vi "SanboxVAlveModbus.vi"() -> ()   [LabVIEW 2019]
uses:
  MB_ENGINE_class/Settings.ctl
  MB_ENGINE_class/Engine State.ctl
  MB_ENGINE_class/Engine Alarms.ctl
  TypeDef/StateValveModbus.ctl
  MB_ENGINE_class/cmd enum.ctl
  ValveModbus_class/ValveModbus.lvclass
  MB_ENGINE_class/MB_ENGINE.lvclass
  D:/H4000/src/modbus engine custom/MB_MODULE_class/MB_MODULE.lvclass
  ValveModbus_class/ValveModbus.lvclass/ValveModbus.ctl
  <vilib>/NI/Modbus Library/API/Wrapper/Create TCP Master.vi
  <vilib>/NI/Modbus Library/API/Wrapper/API Main.lvlib
  MB_MODULE_class/MB_MODULE.lvclass
panel:
  out "StateValveModbus 2":T1
  in  "delta pres":dbl=1.0
  in  "average":i32=10
  in  "ValveModbus":refnum<class "ValveModbus.lvclass">
  in  "milliseconds to wait":u32=300
  out "angle":dbl(graph)=3.4981473129739618
  out "encoder":i32(graph)=72974
  out "step":i32(graph)=124110
  in  "SET":bool
  in  "cmd to write":T2=20 items=["0 Idle"=0, "1 GoTo Absolute Position"=1, "2 GoTo Relative"=2, "10 GoTo Home Position"=10, "11 Set Home Position"=11, "12 Set FindHome Mode"=12, "13 Reset FindHome Mode"=13, "14 Get FindHome State"=14, "20 Hard Stop"=20, "21 HiZ Stop"=21, "22 Soft Stop"=22, "30 Clear Fault"=30, "40 Encoder Set Home"=40, "70 Driver Init"=70]
  out "StateValveModbus":T1
  in  "PRESSURE":dbl(slide)=4.7148288973384025 scale=0.0..10.0
  in  "stop_":bool
  in  "close":bool
  in  "open":bool
  out "dt":u32=10
  in  "cluster 2":T3={"ACC Steps Per Sec^2"=50, "DEC Steps Per Sec^2"=50, "Min Velosity Step Per Sec"=100, "Max Velosity Step Per Sec"=200, "MicroStep"=16}
  out "Numeric":i32=3223
  in  "stop":bool
  out "type":u16=1
  out "Alarms":T4={"OL"=FALSE, "TF"=FALSE, "STL"=FALSE, "OCP"=FALSE, "CPUV"=FALSE, "UVLO"=FALSE, "SPI_ERROR"=FALSE, "Fault"=FALSE, "OL 2"=FALSE, "TF 2"=FALSE, "STL 2"=FALSE, "OCP 2"=FALSE, "CPUV 2"=FALSE, "UVLO 2"=FALSE, "reserved"=TRUE, "InitDone"=TRUE}
  out "Engine State":T5=8 items=["ACCELERATING", "DECELERATINGTOSTOP", "DECELERATING", "STEADY", "INDEX_ACCEL", "NDEX_RUN", "INDEX_DECEL", "INDEX_DWELL", "INACTIVE", "STANDBY", "STANDBYTOINACTIVE"]
  out "RAW Possition":i32=124110
  out "cluster":T3={"ACC Steps Per Sec^2"=100, "DEC Steps Per Sec^2"=100, "Min Velosity Step Per Sec"=100, "Max Velosity Step Per Sec"=200, "MicroStep"=16}
  out "error out":errorcluster
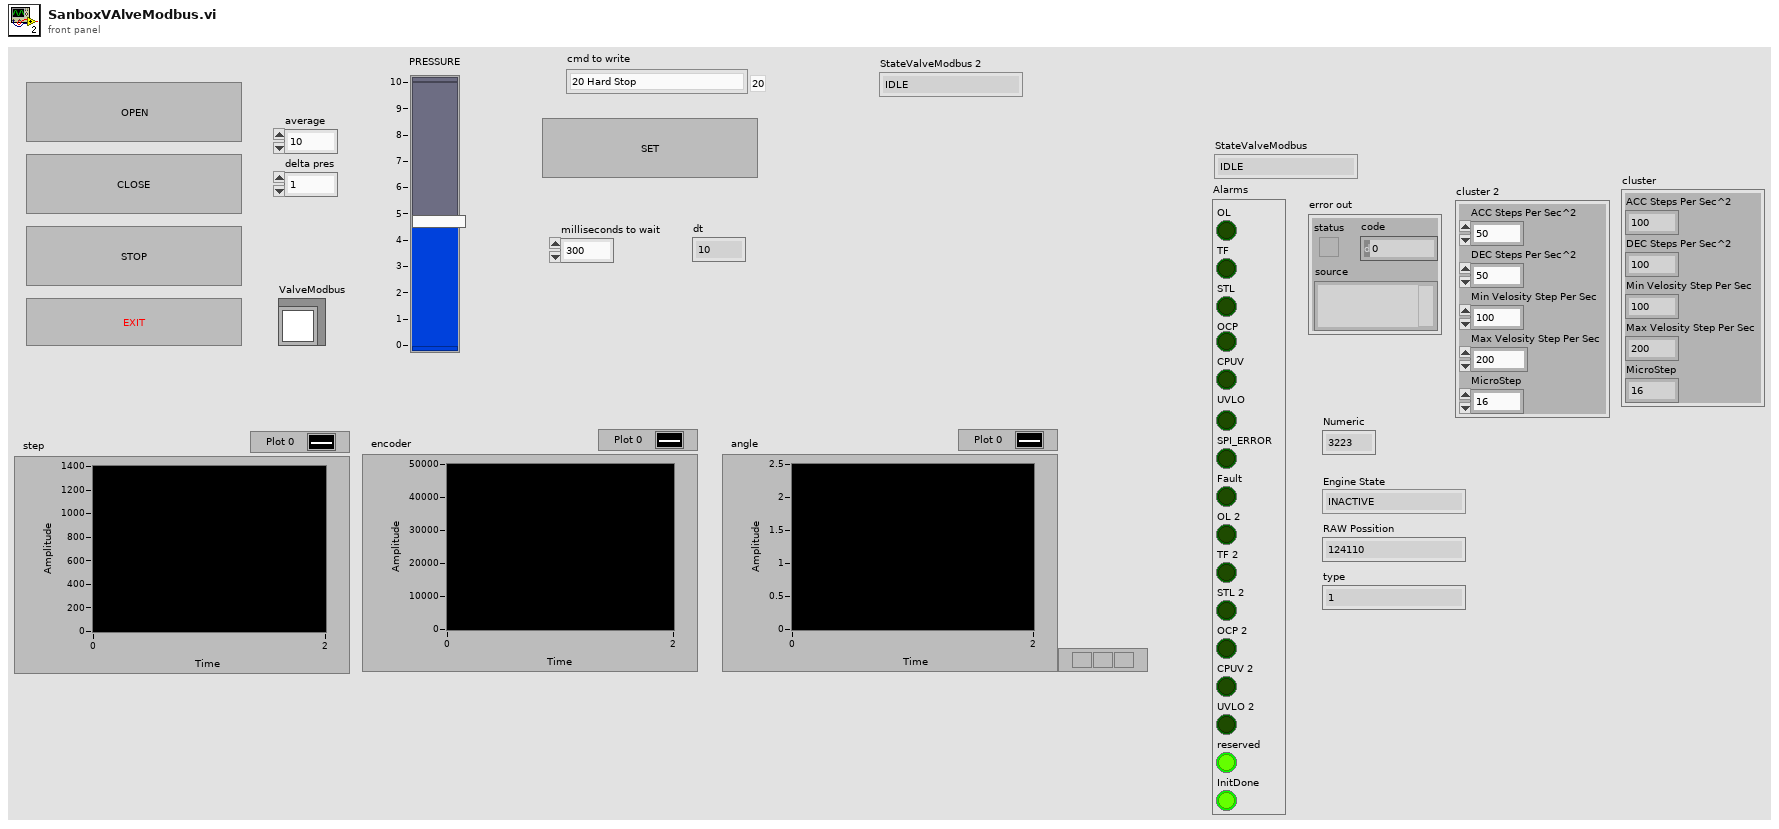
[diagram p1: front panel]
types:
  T1 = typedef "StateValveModbus.ctl" = enum16{"IDLE", "OPEN", "CLOSE", "OPENING", "CLOSING", "STOP"}
  T2 = typedef "MB_ENGINE.lvclass/cmd enum.ctl" = u16
  T3 = typedef "MB_ENGINE.lvclass/Settings.ctl" = cluster{"ACC Steps Per Sec^2":u16, "DEC Steps Per Sec^2":u16, "Min Velosity Step Per Sec":u16, "Max Velosity Step Per Sec":u16, "MicroStep":u16}
  T4 = typedef "MB_ENGINE.lvclass/Engine Alarms.ctl" = cluster{"OL":bool, "TF":bool, "STL":bool, "OCP":bool, "CPUV":bool, "UVLO":bool, "SPI_ERROR":bool, "Fault":bool, "OL 2":bool, "TF 2":bool, "STL 2":bool, "OCP 2":bool, "CPUV 2":bool, "UVLO 2":bool, "reserved":bool, "InitDone":bool}
  T5 = typedef "MB_ENGINE.lvclass/Engine State.ctl" = u16
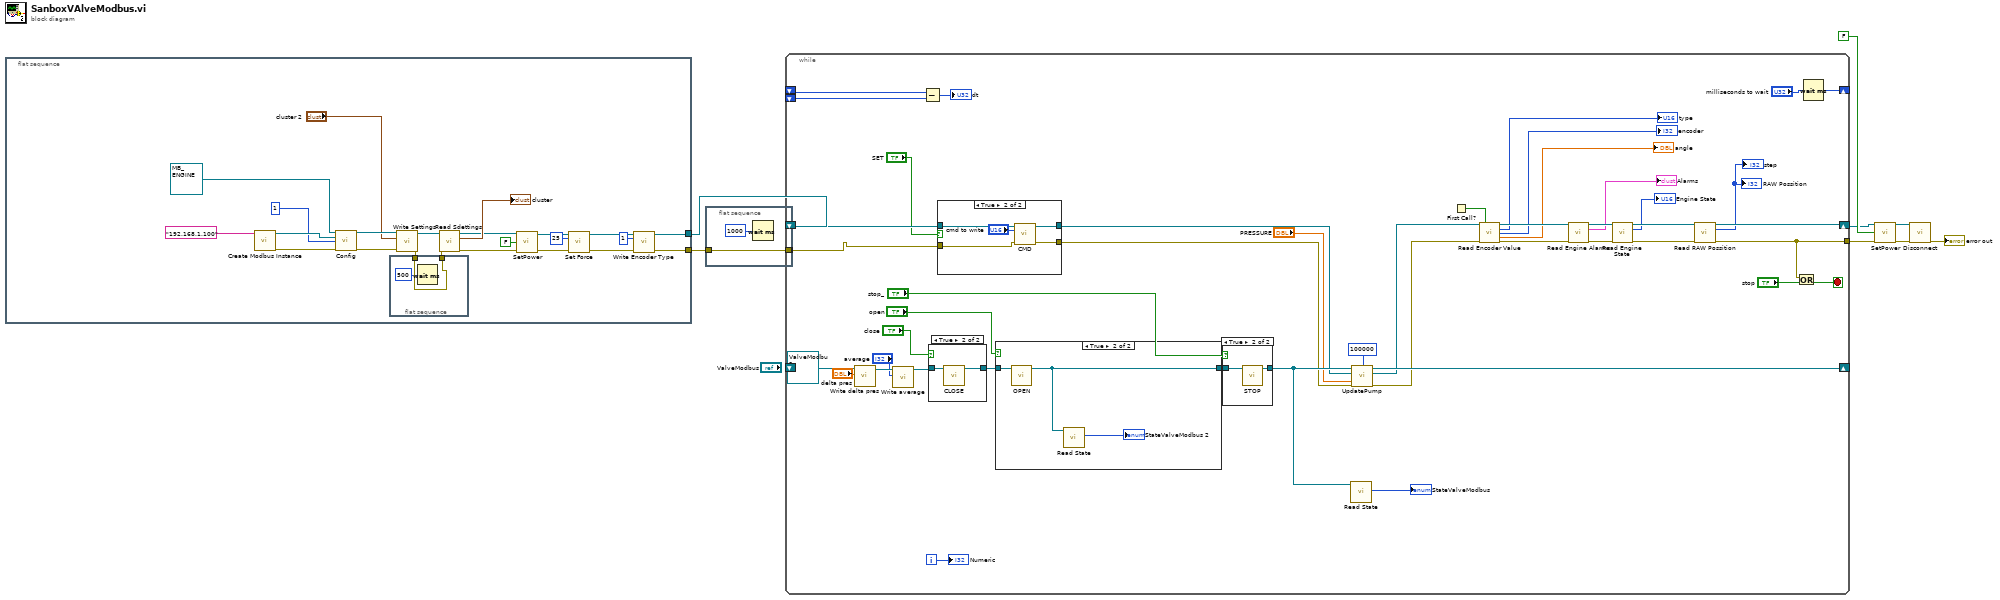
[diagram p0: block diagram]
diagram:
  n1 = flat-sequence {
    tunnel: [w14] -> w9
    tunnel: [w13] -> w2
    frame #0 {
      n2 = call-poly <vilib>:"Create Modbus Instance.vi"("address"="192.168.1.100") -> ("error out"=w30:errorcluster, "TCP master instance"=w32:refnum<class "Modbus Master.lvclass">)  [unwired: 9 in]
      n3 = call-dynamic "Config.vi"("class data in"=refnum<class "MB_ENGINE.lvclass"> refnum ("MB_ENGINE"), "modbus"=w32, "addres"=u16 1, "error in (no error)"=w30) -> ("class data out"=w27:refnum<class "MB_ENGINE.lvclass">, "error out"=w26:errorcluster)  [unwired: 10 in]
      n4 = flat-sequence {
        tunnel: [w35] -> w12
        tunnel: w11 -> [w35]
        frame #0 {
          n5 = Wait (ms)(milliseconds to wait=u32 500) -> ()  [unwired: 1 out]
        }
      }
      n6 = call-dynamic "Write Settings.vi"("class data in"=w27, "cluster"="cluster 2", "error in (no error)"=w26) -> ("class data out"=w24:refnum<class "MB_ENGINE.lvclass">, "error out"=w11:errorcluster)  [unwired: 11 in]
      n7 = call-dynamic "Read Sdettings.vi"("class data in"=w24, "error in (no error)"=w12) -> ("class data out"=w23:refnum<class "MB_ENGINE.lvclass">, "cluster"=→"cluster":T3, "error out"=w22:errorcluster)  [unwired: 11 in]
      n8 = call-dynamic "SetPower.vi"("class data in"=w23, "On"=FALSE, "error in (no error)"=w22) -> ("class data out"=w20:refnum<class "MB_ENGINE.lvclass">, "error out"=w19:errorcluster)  [unwired: 11 in]
      n9 = call-dynamic "Set Force.vi"("class data in"=w20, "percent"=u16 25, "error in (no error)"=w19) -> ("class data out"=w17:refnum<class "MB_ENGINE.lvclass">, "error out"=w16:errorcluster)  [unwired: 11 in]
      n10 = call-dynamic "Write Encoder Type.vi"("class data in"=w17, "U16"=u16 1, "error in (no error)"=w16) -> ("class data out"=w14:refnum<class "MB_ENGINE.lvclass">, "error out"=w13:errorcluster)  [unwired: 11 in]
    }
  }
  n11 = flat-sequence {
    tunnel: [w37] -> w1
    tunnel: w2 -> [w37]
    frame #0 {
      n12 = Wait (ms)(milliseconds to wait=u32 1000) -> ()  [unwired: 1 out]
    }
  }
  n13 = while {
    tunnel: [w76] -> w6
    shift-right: [w73] -> _
    shift-left: _ -> [w72]
    shift-left: _ -> [w71]
    shift-right: [w77] -> w7
    shift-left: w9 -> [w54]
    shift-right: [w60] -> _
    shift-left: refnum<class "ValveModbus.lvclass"> refnum ("ValveModbus") -> [w42]
    tunnel: w1 -> [w43]
    i -> [w75]
    stop <- w78 stop-if-true
    n14 = call "Write delta pres.vi"("delta pres"="delta pres", "ValveModbus in"=w42) -> ("ValveModbus out"=w41:refnum<class "ValveModbus.lvclass">)  [unwired: 9 in]
    n15 = call "Write average.vi"("average"="average", "ValveModbus in"=w41) -> ("ValveModbus out"=w40:refnum<class "ValveModbus.lvclass">)  [unwired: 9 in]
    n16 = Subtract(x=w72, y=w71) -> (x-y=→"dt":u32)
    n17 = case shown="True" "close" {
      tunnel: w40 -> [w97 w99]
      tunnel: [w97 w98] -> w63
      frame False {
      }
      frame True {
        n18 = call "CLOSE.vi"("Pump_1AI_1DO_2DI in"=w99) -> ("Pump_1AI_1DO_2DI out"=w98:refnum<class "ValveModbus.lvclass">)  [unwired: 10 in]
      }
    }
    n19 = case shown="True" "SET" {
      tunnel: w54 -> [w84 w89]
      tunnel: w43 -> [w83 w88]
      tunnel: [w84 w86] -> w53
      tunnel: [w83 w85] -> w52
      frame False {
      }
      frame True {
        n20 = call-dynamic "CMD.vi"("class data in"=w89, "cmd to write"="cmd to write", "error in (no error)"=w88) -> ("class data out"=w86:refnum<class "MB_ENGINE.lvclass">, "error out"=w85:errorcluster)  [unwired: 11 in]
      }
    }
    n21 = case shown="True" "open" {
      tunnel: w63 -> [w93 w96]
      tunnel: [w93 w94] -> w62
      frame False {
      }
      frame True {
        n22 = call "OPEN.vi"("Pump_1AI_1DO_2DI in"=w96) -> ("Pump_1AI_1DO_2DI out"=w94:refnum<class "ValveModbus.lvclass">)  [unwired: 10 in]
        n23 = call "Read State.vi"("Pump_1AI_1DO_2DI in"=w94) -> ("StateValveModbus"=→"StateValveModbus 2":T1)  [unwired: 10 in]
      }
    }
    n24 = case shown="True" "stop_" {
      tunnel: w62 -> [w90 w92]
      tunnel: [w90 w91] -> w61
      frame False {
      }
      frame True {
        n25 = call "STOP.vi"("Pump_1AI_1DO_2DI in"=w92) -> ("Pump_1AI_1DO_2DI out"=w91:refnum<class "ValveModbus.lvclass">)  [unwired: 10 in]
      }
    }
    n26 = call "Read State.vi"("Pump_1AI_1DO_2DI in"=w61) -> ("StateValveModbus"=→"StateValveModbus":T1)  [unwired: 10 in]
    n27 = call "UpdatePump.vi"("Pump_1AI_1DO_2DI in"=w61, "ARG U32"=100000, "MB_ENGINE"=w53, "pressur"="PRESSURE", "error in (no error)"=w52) -> ("Pump_1AI_1DO_2DI out"=w60:refnum<class "ValveModbus.lvclass">, "class data out"=w59:refnum<class "MB_ENGINE.lvclass">, "error out"=w58:errorcluster)  [unwired: 8 in]
    n28 = First Call?() -> (First Call?: T/F=w44:bool)
    n29 = call-dynamic "Read Encoder Value.vi"("class data in"=w59, "init"=w44, "error in (no error)"=w58) -> ("class data out"=w82:refnum<class "MB_ENGINE.lvclass">, "type"=→"type":u16, "Encoder"=→"encoder":i32, "Angel (rad)"=→"angle":dbl, "error out"=w81:errorcluster)  [unwired: 8 in]
    n30 = call-dynamic "Read Engine Alarms.vi"("class data in"=w82, "error in (no error)"=w81) -> ("class data out"=w69:refnum<class "MB_ENGINE.lvclass">, "Alarms"=→"Alarms":T4, "error out"=w67:errorcluster)  [unwired: 11 in]
    n31 = call-dynamic "Read Engine State.vi"("class data in"=w69, "error in (no error)"=w67) -> ("class data out"=w68:refnum<class "MB_ENGINE.lvclass">, "Engine State"=→"Engine State":T5, "error out"=w66:errorcluster)  [unwired: 11 in]
    n32 = call-dynamic "Read RAW Possition.vi"("class data in"=w68, "error in (no error)"=w66) -> ("class data out"=w77:refnum<class "MB_ENGINE.lvclass">, "RAW Possition"=→"RAW Possition" →"step":i32, "error out"=w76:errorcluster)  [unwired: 11 in]
    n33 = Or(x=w76, y="stop") -> (x .or. y?=w78:bool)
    n34 = Wait (ms)(milliseconds to wait="milliseconds to wait") -> (millisecond timer value=w73:u32)
    "Numeric" <- w75
  }
  n35 = call-dynamic "SetPower.vi"("class data in"=w7, "On"=FALSE, "error in (no error)"=w6) -> ("class data out"=w4:refnum<class "MB_ENGINE.lvclass">, "error out"=w5:errorcluster)  [unwired: 11 in]
  n36 = call "Disconnect.vi"("MB_MODULE"=w4, "error in"=w5) -> ("error out"=→"error out":errorcluster)  [unwired: 13 in]
